vi "uTTA_SetDUT_Name.vi"(8 "error in":errorcluster, 10 "DUT Name":string, 11 "VISA Refnum in":refnum<visa-resource-name>) -> (0 "error out":errorcluster, 2 "Received":string, 3 "VISA Refnum out":refnum<visa-resource-name>)   [LabVIEW 2021]
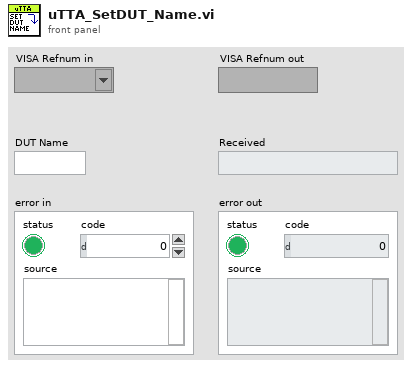
[diagram p1: front panel]
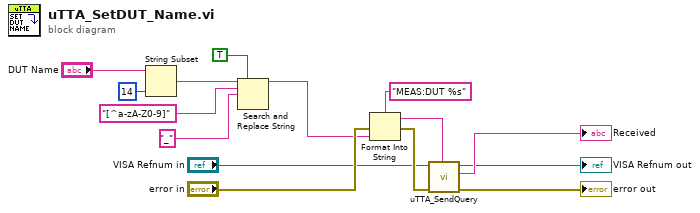
[diagram p0: block diagram]
diagram:
  n1 = String Subset(string="DUT Name", length (rest)=14 ("length (rest)")) -> (substring=w2:string)  [unwired: 1 in]
  n2 = Search and Replace String(replace all?=TRUE ("replace all? (F)"), input string=w2, search string="[^a-zA-Z0-9]", replace string="_" ("replace string (\"\")")) -> (result string=w1:string)  [unwired: 4 in, 3 out]
  n3 = Format Into String(format string="MEAS:DUT %s", error in="error in", w1) -> (resulting string=w12:string, error out=w14:errorcluster)  [unwired: 1 in]
  n4 = call "uTTA_SendQuery.vi"("Send String"=w12, "error in (no error)"=w14, "VISA Refnum in"="VISA Refnum in") -> ("error out"=→"error out":errorcluster, "Received"=→"Received":string, "VISA Refnum out"=→"VISA Refnum out":refnum<visa-resource-name>)  [unwired: 6 in]
